vi "WriteTCSInfo.vi"(4 "error in (no error)":errorcluster, 5 "# of Entries (before)":i16, 6 "TCSInfo":T1, 7 "Pathto FITS Header File":path) -> (0 "error out":errorcluster, 2 "# of Entries (after)":i16, 3 "Path to FITS Header File":path)   [LabVIEW 2015]
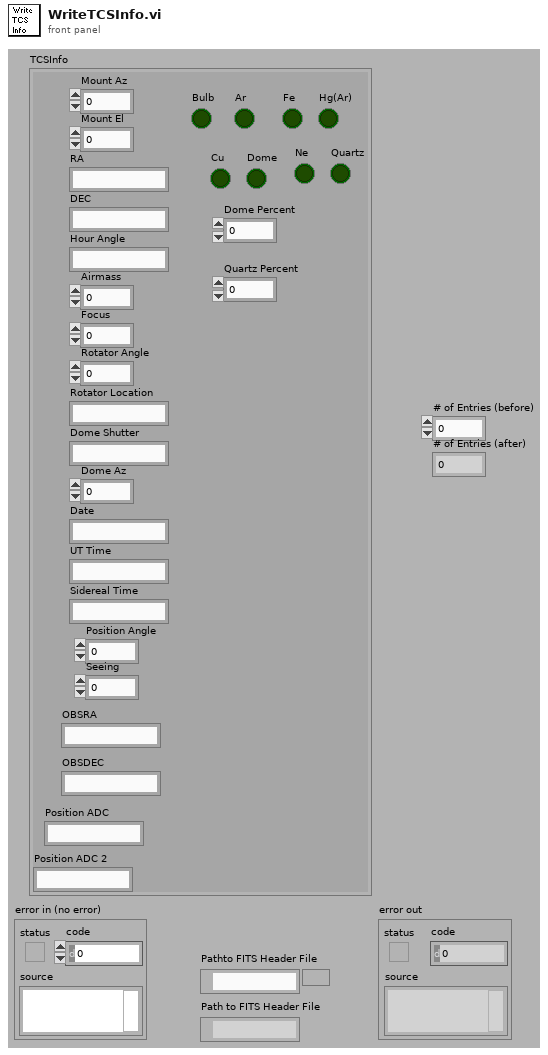
[diagram p1: front panel]
types:
  T1 = cluster{"Mount Az":dbl, "Mount El":dbl, "RA":string, "DEC":string, "Hour Angle":string, "Airmass":dbl, "Focus":dbl, "Rotator Angle":dbl, "Rotator Location":string, "Dome Shutter":string, "Dome Az":dbl, "Date":string, "UT Time":string, "Sidereal Time":string, "Position Angle":dbl, "Seeing":dbl, "OBSRA":string, "OBSDEC":string, "Position ADC":string, "Position ADC 2":string, "Bulb":bool, "Ar":bool, "Cu":bool, "Dome":bool, "Fe":bool, "Hg(Ar)":bool, "Ne":bool, "Quartz":bool, "Dome Percent":dbl, "Quartz Percent":dbl}
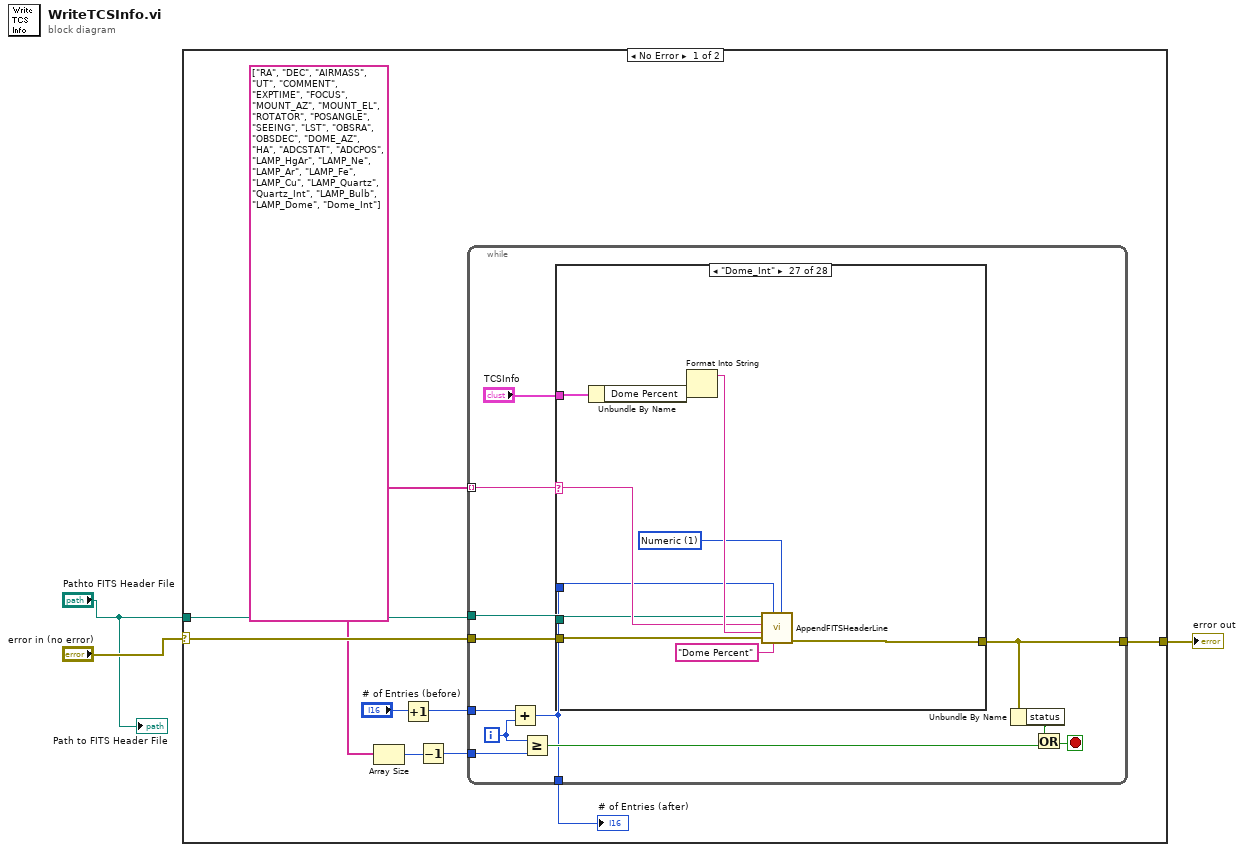
[diagram p0: block diagram]
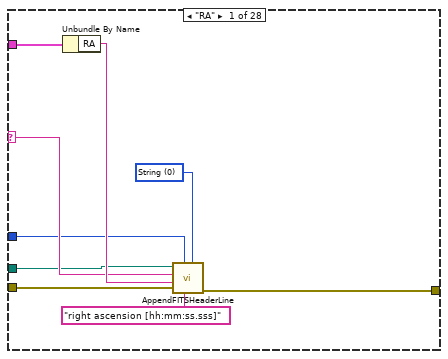
[diagram p2: hidden frame]
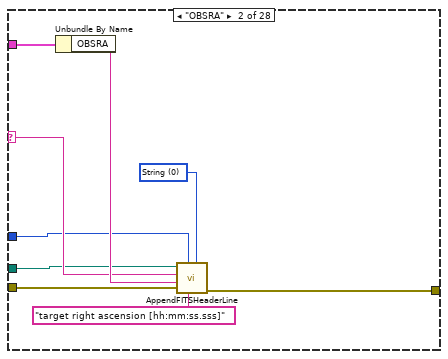
[diagram p3: hidden frame]
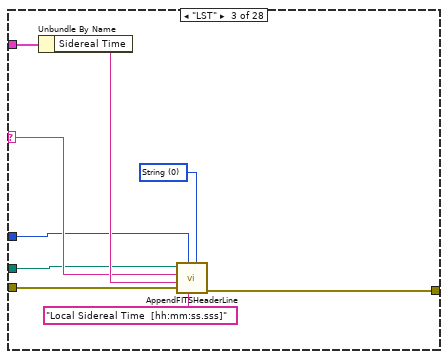
[diagram p4: hidden frame]
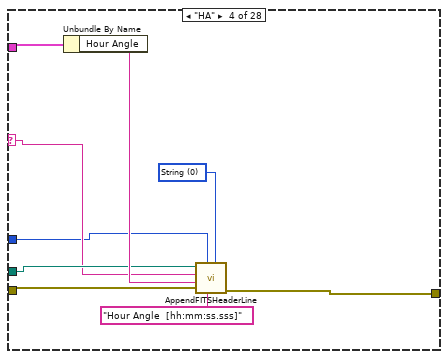
[diagram p5: hidden frame]
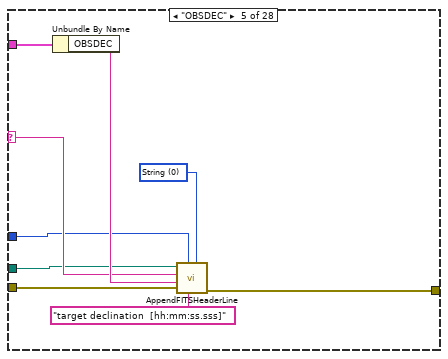
[diagram p6: hidden frame]
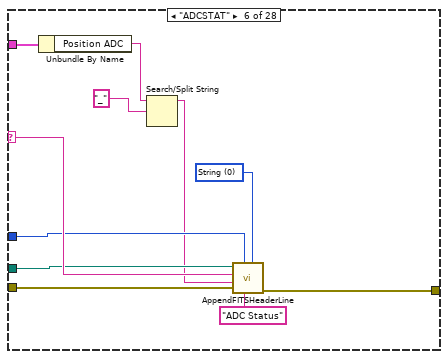
[diagram p7: hidden frame]
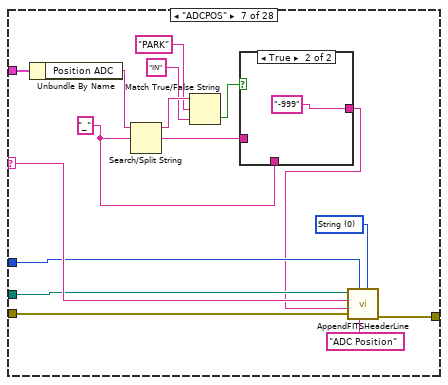
[diagram p8: hidden frame]
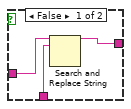
[diagram p9: hidden frame]
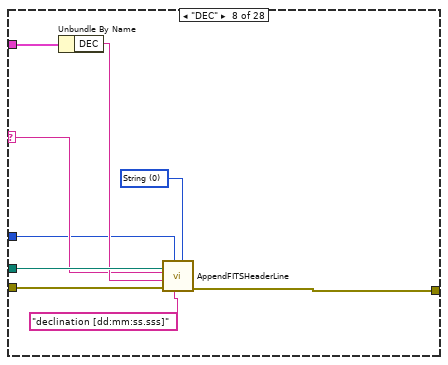
[diagram p10: hidden frame]
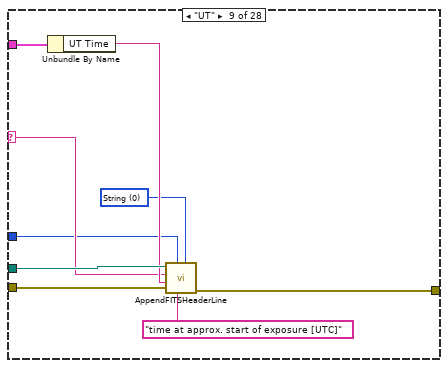
[diagram p11: hidden frame]
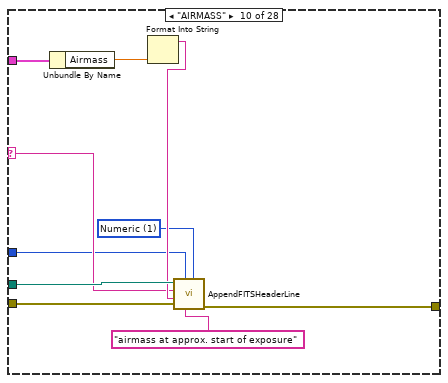
[diagram p12: hidden frame]
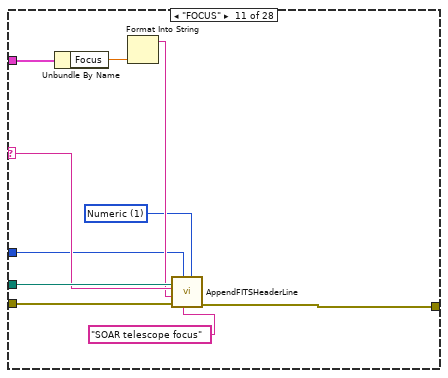
[diagram p13: hidden frame]
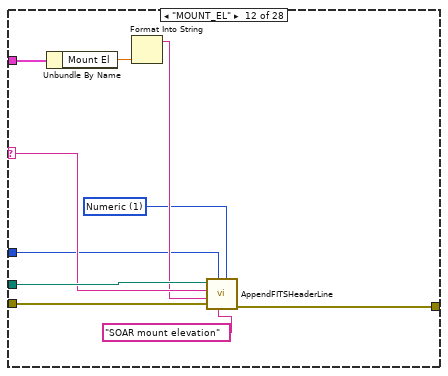
[diagram p14: hidden frame]
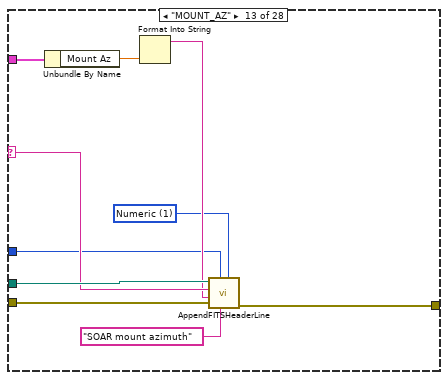
[diagram p15: hidden frame]
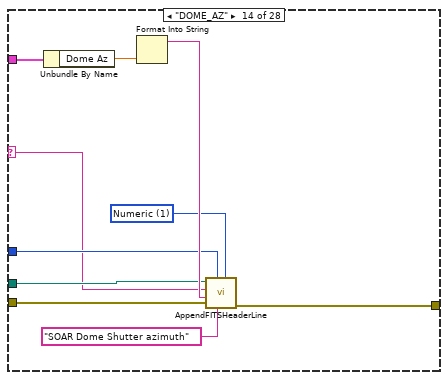
[diagram p16: hidden frame]
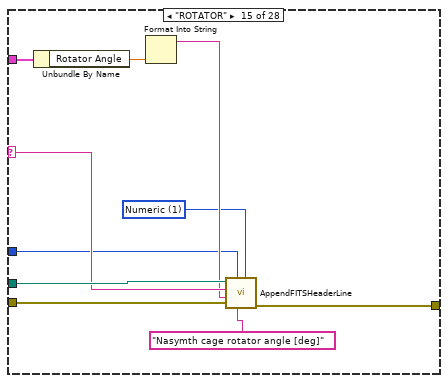
[diagram p17: hidden frame]
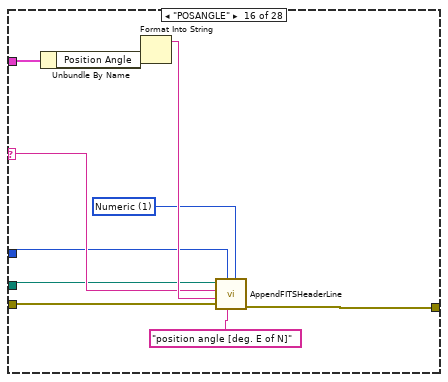
[diagram p18: hidden frame]
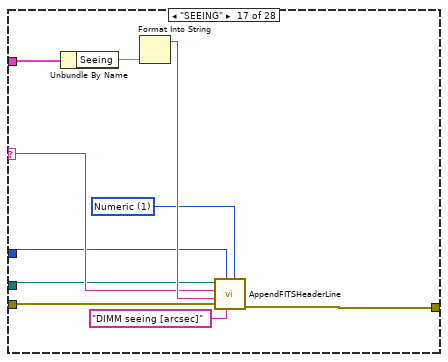
[diagram p19: hidden frame]
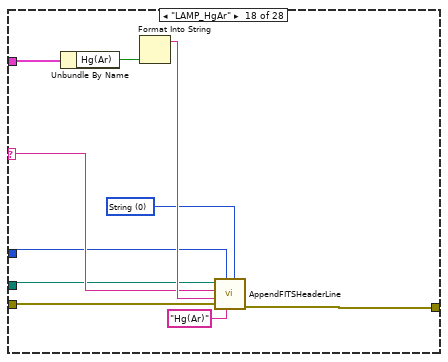
[diagram p20: hidden frame]
diagram:
  n1 = case shown="No Error" "error in (no error)" {
    selector: "error in (no error)" -> [w12 w300]
    tunnel: [w8 w300] -> w2
    tunnel: "Pathto FITS Header File" -> [w7 _]
    frame No Error {
      w11 = string[] ["RA", "DEC", "AIRMASS", "UT", "COMMENT", "EXPTIME", "FOCUS", "MOUNT_AZ", "MOUNT_EL", "ROTATOR", "POSANGLE", "SEEING", "LST", "OBSRA", "OBSDEC", "DOME_AZ", "HA", "ADCSTAT", "ADCPOS", "LAMP_HgAr", "LAMP_Ne", "LAMP_Ar", "LAMP_Fe", "LAMP_Cu", "LAMP_Quartz", "Quartz_Int", "LAMP_Bulb", "LAMP_Dome", "Dome_Int"]
      n2 = Array Size(array=w11) -> (size(s)=w10:i32)
      n3 = Increment(x="# of Entries (before)") -> (x+1=w5:i16)
      n4 = Decrement(x=w10) -> (x-1=w9:i32)
      n5 = while {
        tunnel: w12 -> [w24]
        tunnel: w11 -> [w21] mode=indexing
        tunnel: w9 -> [w20]
        tunnel: [w19] -> w8
        tunnel: w7 -> [w16]
        tunnel: w5 -> [w14]
        tunnel: [w13] -> w4
        i -> [w15]
        stop <- w23 stop-if-true
        n6 = Add(x=w14, y=w15) -> (x+y=w13:i32)
        n7 = Greater Or Equal?(x=w15, y=w20) -> (x >= y?=w18:bool)
        n8 = case shown="\"Dome_Int\"" w21 {
          selector: w21 -> [w29 w38 w47 w54 w65 w77 w93 w104 w113 w122 w134 w143 w153 w160 w173 w184 w194 w204 w214 w224 w234 w244 w254 w264 w274 w284 w294 _]
          tunnel: w24 -> [w32 w35 w44 w56 w62 w74 w90 w108 w117 w126 w137 w146 w156 w163 w176 w181 w191 w201 w211 w221 w231 w241 w251 w261 w271 w281 w291 w299]
          tunnel: [w31 w34 w43 w57 w61 w73 w89 w107 w116 w125 w136 w145 w155 w164 w175 w180 w190 w200 w210 w220 w230 w240 w250 w260 w270 w280 w290 w299] -> w19
          tunnel: "TCSInfo" -> [w33 w39 w48 w52 w66 w78 w94 w109 w118 w128 w138 w148 w158 w159 w178 w185 w195 w205 w215 w225 w235 w245 w255 w265 w275 w285 w295 _]
          tunnel: w16 -> [w28 w36 w45 w55 w63 w75 w91 w106 w115 w124 w135 w144 w154 w162 w174 w182 w192 w202 w212 w222 w232 w242 w252 w262 w272 w282 w292 _]
          tunnel: w13 -> [w27 w37 w46 w53 w64 w76 w92 w103 w112 w121 w131 w140 w151 w161 w171 w183 w193 w203 w213 w223 w233 w243 w253 w263 w273 w283 w293 _]
          frame "RA" {
            w26 = u16 0 items=["String", "Numeric", "Boolean"] ("Entry Type")
            n9 = Unbundle By Name(w33) -> ("RA"=w30:string)
            n10 = call "AppendFITSHeaderLine.vi"("Entry Type"=w26, "Comment"="right ascension [hh:mm:ss.sss]", "Entry #"=w27, "error in (no error)"=w32, "Element Value"=w30, "Element Name"=w29, "file path (dialog if empty)"=w28) -> ("error out"=w31:errorcluster)  [unwired: 3 in]
          }
          frame "OBSRA" {
            w41 = u16 0 items=["String", "Numeric", "Boolean"] ("Entry Type")
            n11 = Unbundle By Name(w39) -> ("OBSRA"=w42:string)
            n12 = call "AppendFITSHeaderLine.vi"("Entry Type"=w41, "Comment"="target right ascension [hh:mm:ss.sss]", "Entry #"=w37, "error in (no error)"=w35, "Element Value"=w42, "Element Name"=w38, "file path (dialog if empty)"=w36) -> ("error out"=w34:errorcluster)  [unwired: 3 in]
          }
          frame "LST" {
            w50 = u16 0 items=["String", "Numeric", "Boolean"] ("Entry Type")
            n13 = Unbundle By Name(w48) -> ("Sidereal Time"=w51:string)
            n14 = call "AppendFITSHeaderLine.vi"("Entry Type"=w50, "Comment"="Local Sidereal Time  [hh:mm:ss.sss]", "Entry #"=w46, "error in (no error)"=w44, "Element Value"=w51, "Element Name"=w47, "file path (dialog if empty)"=w45) -> ("error out"=w43:errorcluster)  [unwired: 3 in]
          }
          frame "HA" {
            w59 = u16 0 items=["String", "Numeric", "Boolean"] ("Entry Type")
            n15 = Unbundle By Name(w52) -> ("Hour Angle"=w60:string)
            n16 = call "AppendFITSHeaderLine.vi"("Entry Type"=w59, "Comment"="Hour Angle  [hh:mm:ss.sss]", "Entry #"=w53, "error in (no error)"=w56, "Element Value"=w60, "Element Name"=w54, "file path (dialog if empty)"=w55) -> ("error out"=w57:errorcluster)  [unwired: 3 in]
          }
          frame "OBSDEC" {
            w68 = u16 0 items=["String", "Numeric", "Boolean"] ("Entry Type")
            n17 = Unbundle By Name(w66) -> ("OBSDEC"=w69:string)
            n18 = call "AppendFITSHeaderLine.vi"("Entry Type"=w68, "Comment"="target declination  [hh:mm:ss.sss]", "Entry #"=w64, "error in (no error)"=w62, "Element Value"=w69, "Element Name"=w65, "file path (dialog if empty)"=w63) -> ("error out"=w61:errorcluster)  [unwired: 3 in]
          }
          frame "ADCSTAT" {
            w80 = u16 0 items=["String", "Numeric", "Boolean"] ("Entry Type")
            n19 = Unbundle By Name(w78) -> ("Position ADC"=w72:string)
            n20 = Search/Split String(string=w72, search string/char (-)="_" ("Comment")) -> (substring before match=w70:string)  [unwired: 1 in, 2 out]
            n21 = call "AppendFITSHeaderLine.vi"("Entry Type"=w80, "Comment"="ADC Status", "Entry #"=w76, "error in (no error)"=w74, "Element Value"=w70, "Element Name"=w77, "file path (dialog if empty)"=w75) -> ("error out"=w73:errorcluster)  [unwired: 3 in]
          }
          frame "ADCPOS" {
            w96 = u16 0 items=["String", "Numeric", "Boolean"] ("Entry Type")
            w83 = "_" ("Comment")
            n22 = Unbundle By Name(w94) -> ("Position ADC"=w88:string)
            n23 = Search/Split String(string=w88, search string/char (-)=w83) -> (substring before match=w87:string, match + rest of string=w84:string)  [unwired: 1 in, 1 out]
            n24 = Match True/False String(2:"IN" ("Comment"), 3:"PARK" ("Comment"), 4:w87) -> (0:w85:bool)  [unwired: 1 out]
            n25 = case shown="True" w85 {
              tunnel: w84 -> [w99 _]
              tunnel: w83 -> [w98 _]
              tunnel: [w97 "-999" ("Comment")] -> w82
              frame False {
                n26 = Search and Replace String(input string=w99, search string=w98) -> (result string=w97:string)  [unwired: 6 in, 3 out]
              }
              frame True {
              }
            }
            n27 = call "AppendFITSHeaderLine.vi"("Entry Type"=w96, "Comment"="ADC Position", "Entry #"=w92, "error in (no error)"=w90, "Element Value"=w82, "Element Name"=w93, "file path (dialog if empty)"=w91) -> ("error out"=w89:errorcluster)  [unwired: 3 in]
          }
          frame "DEC" {
            w102 = u16 0 items=["String", "Numeric", "Boolean"] ("Entry Type")
            n28 = Unbundle By Name(w109) -> ("DEC"=w105:string)
            n29 = call "AppendFITSHeaderLine.vi"("Entry Type"=w102, "Comment"="declination [dd:mm:ss.sss]", "Entry #"=w103, "error in (no error)"=w108, "Element Value"=w105, "Element Name"=w104, "file path (dialog if empty)"=w106) -> ("error out"=w107:errorcluster)  [unwired: 3 in]
          }
          frame "UT" {
            w111 = u16 0 items=["String", "Numeric", "Boolean"] ("Entry Type")
            n30 = Unbundle By Name(w118) -> ("UT Time"=w114:string)
            n31 = call "AppendFITSHeaderLine.vi"("Entry Type"=w111, "Comment"="time at approx. start of exposure [UTC]", "Entry #"=w112, "error in (no error)"=w117, "Element Value"=w114, "Element Name"=w113, "file path (dialog if empty)"=w115) -> ("error out"=w116:errorcluster)  [unwired: 3 in]
          }
          frame "AIRMASS" {
            w120 = u16 1 items=["String", "Numeric", "Boolean"] ("Entry Type")
            n32 = Unbundle By Name(w128) -> ("Airmass"=w127:dbl)
            n33 = Format Into String(w127) -> (resulting string=w123:string)  [unwired: 3 in, 1 out]
            n34 = call "AppendFITSHeaderLine.vi"("Entry Type"=w120, "Comment"="airmass at approx. start of exposure", "Entry #"=w121, "error in (no error)"=w126, "Element Value"=w123, "Element Name"=w122, "file path (dialog if empty)"=w124) -> ("error out"=w125:errorcluster)  [unwired: 3 in]
          }
          frame "FOCUS" {
            w130 = u16 1 items=["String", "Numeric", "Boolean"] ("Entry Type")
            n35 = Unbundle By Name(w138) -> ("Focus"=w133:dbl)
            n36 = Format Into String(w133) -> (resulting string=w132:string)  [unwired: 3 in, 1 out]
            n37 = call "AppendFITSHeaderLine.vi"("Entry Type"=w130, "Comment"="SOAR telescope focus", "Entry #"=w131, "error in (no error)"=w137, "Element Value"=w132, "Element Name"=w134, "file path (dialog if empty)"=w135) -> ("error out"=w136:errorcluster)  [unwired: 3 in]
          }
          frame "MOUNT_EL" {
            w141 = u16 1 items=["String", "Numeric", "Boolean"] ("Entry Type")
            n38 = Unbundle By Name(w148) -> ("Mount El"=w147:dbl)
            n39 = Format Into String(w147) -> (resulting string=w142:string)  [unwired: 3 in, 1 out]
            n40 = call "AppendFITSHeaderLine.vi"("Entry Type"=w141, "Comment"="SOAR mount elevation", "Entry #"=w140, "error in (no error)"=w146, "Element Value"=w142, "Element Name"=w143, "file path (dialog if empty)"=w144) -> ("error out"=w145:errorcluster)  [unwired: 3 in]
          }
          frame "MOUNT_AZ" {
            w150 = u16 1 items=["String", "Numeric", "Boolean"] ("Entry Type")
            n41 = Unbundle By Name(w158) -> ("Mount Az"=w157:dbl)
            n42 = Format Into String(w157) -> (resulting string=w152:string)  [unwired: 3 in, 1 out]
            n43 = call "AppendFITSHeaderLine.vi"("Entry Type"=w150, "Comment"="SOAR mount azimuth", "Entry #"=w151, "error in (no error)"=w156, "Element Value"=w152, "Element Name"=w153, "file path (dialog if empty)"=w154) -> ("error out"=w155:errorcluster)  [unwired: 3 in]
          }
          frame "DOME_AZ" {
            w166 = u16 1 items=["String", "Numeric", "Boolean"] ("Entry Type")
            n44 = Unbundle By Name(w159) -> ("Dome Az"=w168:dbl)
            n45 = Format Into String(w168) -> (resulting string=w167:string)  [unwired: 3 in, 1 out]
            n46 = call "AppendFITSHeaderLine.vi"("Entry Type"=w166, "Comment"="SOAR Dome Shutter azimuth", "Entry #"=w161, "error in (no error)"=w163, "Element Value"=w167, "Element Name"=w160, "file path (dialog if empty)"=w162) -> ("error out"=w164:errorcluster)  [unwired: 3 in]
          }
          frame "ROTATOR" {
            w170 = u16 1 items=["String", "Numeric", "Boolean"] ("Entry Type")
            n47 = Unbundle By Name(w178) -> ("Rotator Angle"=w177:dbl)
            n48 = Format Into String(w177) -> (resulting string=w172:string)  [unwired: 3 in, 1 out]
            n49 = call "AppendFITSHeaderLine.vi"("Entry Type"=w170, "Comment"="Nasymth cage rotator angle [deg]", "Entry #"=w171, "error in (no error)"=w176, "Element Value"=w172, "Element Name"=w173, "file path (dialog if empty)"=w174) -> ("error out"=w175:errorcluster)  [unwired: 3 in]
          }
          frame "POSANGLE" {
            w186 = u16 1 items=["String", "Numeric", "Boolean"] ("Entry Type")
            n50 = Unbundle By Name(w185) -> ("Position Angle"=w188:dbl)
            n51 = Format Into String(w188) -> (resulting string=w187:string)  [unwired: 3 in, 1 out]
            n52 = call "AppendFITSHeaderLine.vi"("Entry Type"=w186, "Comment"="position angle [deg. E of N]", "Entry #"=w183, "error in (no error)"=w181, "Element Value"=w187, "Element Name"=w184, "file path (dialog if empty)"=w182) -> ("error out"=w180:errorcluster)  [unwired: 3 in]
          }
          frame "SEEING" {
            w196 = u16 1 items=["String", "Numeric", "Boolean"] ("Entry Type")
            n53 = Unbundle By Name(w195) -> ("Seeing"=w198:dbl)
            n54 = Format Into String(w198) -> (resulting string=w197:string)  [unwired: 3 in, 1 out]
            n55 = call "AppendFITSHeaderLine.vi"("Entry Type"=w196, "Comment"="DIMM seeing [arcsec]", "Entry #"=w193, "error in (no error)"=w191, "Element Value"=w197, "Element Name"=w194, "file path (dialog if empty)"=w192) -> ("error out"=w190:errorcluster)  [unwired: 3 in]
          }
          frame "LAMP_HgAr" {
            w206 = u16 0 items=["String", "Numeric", "Boolean"] ("Entry Type")
            n56 = Unbundle By Name(w205) -> ("Hg(Ar)"=w208:bool)
            n57 = Format Into String(w208) -> (resulting string=w207:string)  [unwired: 3 in, 1 out]
            n58 = call "AppendFITSHeaderLine.vi"("Entry Type"=w206, "Comment"="Hg(Ar)", "Entry #"=w203, "error in (no error)"=w201, "Element Value"=w207, "Element Name"=w204, "file path (dialog if empty)"=w202) -> ("error out"=w200:errorcluster)  [unwired: 3 in]
          }
          frame "LAMP_Ne" {
            w216 = u16 0 items=["String", "Numeric", "Boolean"] ("Entry Type")
            n59 = Unbundle By Name(w215) -> ("Ne"=w218:bool)
            n60 = Format Into String(w218) -> (resulting string=w217:string)  [unwired: 3 in, 1 out]
            n61 = call "AppendFITSHeaderLine.vi"("Entry Type"=w216, "Comment"="Neon", "Entry #"=w213, "error in (no error)"=w211, "Element Value"=w217, "Element Name"=w214, "file path (dialog if empty)"=w212) -> ("error out"=w210:errorcluster)  [unwired: 3 in]
          }
          frame "LAMP_Ar" {
            w226 = u16 0 items=["String", "Numeric", "Boolean"] ("Entry Type")
            n62 = Unbundle By Name(w225) -> ("Ar"=w228:bool)
            n63 = Format Into String(w228) -> (resulting string=w227:string)  [unwired: 3 in, 1 out]
            n64 = call "AppendFITSHeaderLine.vi"("Entry Type"=w226, "Comment"="Argon", "Entry #"=w223, "error in (no error)"=w221, "Element Value"=w227, "Element Name"=w224, "file path (dialog if empty)"=w222) -> ("error out"=w220:errorcluster)  [unwired: 3 in]
          }
          frame "LAMP_Fe" {
            w236 = u16 0 items=["String", "Numeric", "Boolean"] ("Entry Type")
            n65 = Unbundle By Name(w235) -> ("Fe"=w238:bool)
            n66 = Format Into String(w238) -> (resulting string=w237:string)  [unwired: 3 in, 1 out]
            n67 = call "AppendFITSHeaderLine.vi"("Entry Type"=w236, "Comment"="Iron", "Entry #"=w233, "error in (no error)"=w231, "Element Value"=w237, "Element Name"=w234, "file path (dialog if empty)"=w232) -> ("error out"=w230:errorcluster)  [unwired: 3 in]
          }
          frame "LAMP_Cu" {
            w246 = u16 0 items=["String", "Numeric", "Boolean"] ("Entry Type")
            n68 = Unbundle By Name(w245) -> ("Cu"=w248:bool)
            n69 = Format Into String(w248) -> (resulting string=w247:string)  [unwired: 3 in, 1 out]
            n70 = call "AppendFITSHeaderLine.vi"("Entry Type"=w246, "Comment"="Copper", "Entry #"=w243, "error in (no error)"=w241, "Element Value"=w247, "Element Name"=w244, "file path (dialog if empty)"=w242) -> ("error out"=w240:errorcluster)  [unwired: 3 in]
          }
          frame "LAMP_Quartz" {
            w256 = u16 0 items=["String", "Numeric", "Boolean"] ("Entry Type")
            n71 = Unbundle By Name(w255) -> ("Quartz"=w258:bool)
            n72 = Format Into String(w258) -> (resulting string=w257:string)  [unwired: 3 in, 1 out]
            n73 = call "AppendFITSHeaderLine.vi"("Entry Type"=w256, "Comment"="Quartz", "Entry #"=w253, "error in (no error)"=w251, "Element Value"=w257, "Element Name"=w254, "file path (dialog if empty)"=w252) -> ("error out"=w250:errorcluster)  [unwired: 3 in]
          }
          frame "Quartz_Int" {
            w266 = u16 1 items=["String", "Numeric", "Boolean"] ("Entry Type")
            n74 = Unbundle By Name(w265) -> ("Quartz Percent"=w268:dbl)
            n75 = Format Into String(w268) -> (resulting string=w267:string)  [unwired: 3 in, 1 out]
            n76 = call "AppendFITSHeaderLine.vi"("Entry Type"=w266, "Comment"="Quartz Percent", "Entry #"=w263, "error in (no error)"=w261, "Element Value"=w267, "Element Name"=w264, "file path (dialog if empty)"=w262) -> ("error out"=w260:errorcluster)  [unwired: 3 in]
          }
          frame "LAMP_Bulb" {
            w276 = u16 0 items=["String", "Numeric", "Boolean"] ("Entry Type")
            n77 = Unbundle By Name(w275) -> ("Bulb"=w278:bool)
            n78 = Format Into String(w278) -> (resulting string=w277:string)  [unwired: 3 in, 1 out]
            n79 = call "AppendFITSHeaderLine.vi"("Entry Type"=w276, "Comment"="Bulb", "Entry #"=w273, "error in (no error)"=w271, "Element Value"=w277, "Element Name"=w274, "file path (dialog if empty)"=w272) -> ("error out"=w270:errorcluster)  [unwired: 3 in]
          }
          frame "LAMP_Dome" {
            w286 = u16 0 items=["String", "Numeric", "Boolean"] ("Entry Type")
            n80 = Unbundle By Name(w285) -> ("Dome"=w288:bool)
            n81 = Format Into String(w288) -> (resulting string=w287:string)  [unwired: 3 in, 1 out]
            n82 = call "AppendFITSHeaderLine.vi"("Entry Type"=w286, "Comment"="Dome", "Entry #"=w283, "error in (no error)"=w281, "Element Value"=w287, "Element Name"=w284, "file path (dialog if empty)"=w282) -> ("error out"=w280:errorcluster)  [unwired: 3 in]
          }
          frame "Dome_Int" {
            w296 = u16 1 items=["String", "Numeric", "Boolean"] ("Entry Type")
            n83 = Unbundle By Name(w295) -> ("Dome Percent"=w298:dbl)
            n84 = Format Into String(w298) -> (resulting string=w297:string)  [unwired: 3 in, 1 out]
            n85 = call "AppendFITSHeaderLine.vi"("Entry Type"=w296, "Comment"="Dome Percent", "Entry #"=w293, "error in (no error)"=w291, "Element Value"=w297, "Element Name"=w294, "file path (dialog if empty)"=w292) -> ("error out"=w290:errorcluster)  [unwired: 3 in]
          }
          frame "", Default {
          }
        }
        n86 = Unbundle By Name(w19) -> ("status"=w17:bool)
        n87 = Or(x=w17, y=w18) -> (x .or. y?=w23:bool)
      }
      "# of Entries (after)" <- w4
    }
    frame Error {
    }
  }
  "error out" <- w2
  "Path to FITS Header File" <- "Pathto FITS Header File"
